vi "Start Module.vi"(8 "error in (no error)":errorcluster, 10 "Config Section":string, 11 "Run as Singleton? (F)":bool) -> (0 "error out":errorcluster, 1 "Wait for Event Sync?":bool, 2 "DB_CONNECTOR Broadcast Events":T1, 3 "Module ID":i32)   [LabVIEW 2014, in "DB_CONNECTOR.lvlib"]
doc: "Launches the Module Main.vi.\n_____\nBased on Delacor QMH Project Template 4.0.0.43."
uses:
  DB_CONNECTOR.lvlib
  Broadcast Events--cluster.ctl
  Did Init Argument--cluster.ctl
  Status Updated Argument--cluster.ctl
  Error Reported Argument--cluster.ctl
  Stop Argument--cluster.ctl
  Get Module Execution Status Argument--cluster.ctl
  Fast Query Reply Argument--cluster.ctl
  Module Running State--enum.ctl
  <vilib>/Delacor/Delacor QMH/Libraries/Cloneable Module Admin_class/Delacor_lib_QMH_Cloneable Module Admin.lvclass
  <vilib>/Delacor/Delacor QMH/Libraries/Cloneable Module Admin_class/Delacor_lib_QMH_Cloneable Module Admin.lvclass/Delacor_lib_QMH_Cloneable Module Admin.ctl
  <vilib>/Delacor/Delacor QMH/Libraries/Module Admin_class/Delacor_lib_QMH_Module Admin.lvclass/Delacor_lib_QMH_Module Admin.ctl
  <vilib>/Delacor/Delacor QMH/Libraries/Cloneable Module Admin_class/Delacor_lib_QMH_Set Module ID.vi
  <vilib>/Delacor/Delacor QMH/Libraries/Module Admin_class/Delacor_lib_QMH_Set External Launch.vi
  <vilib>/Utility/error.llb/Error Cluster From Error Code.vi
  <vilib>/ErrorRing/Error Ring.xnode
  Clone Registration/Clone Registration.lvlib
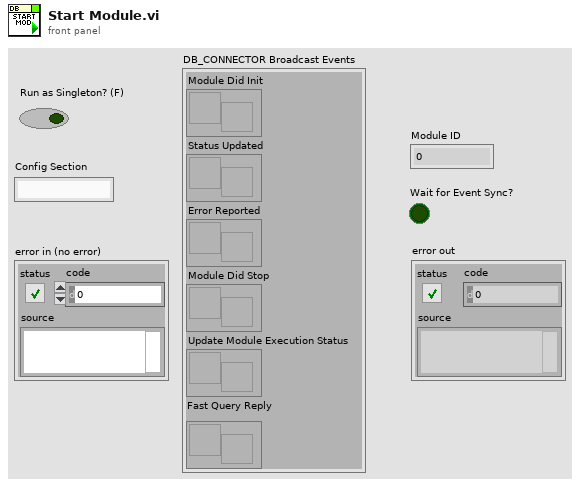
[diagram p1: front panel]
types:
  T1 = typedef "DB_CONNECTOR.lvlib/Broadcast Events--cluster.ctl" = cluster{"Module Did Init":refnum<user-event>, "Status Updated":refnum<user-event>, "Error Reported":refnum<user-event>, "Module Did Stop":refnum<user-event>, "Update Module Execution Status":refnum<user-event>, "Fast Query Reply":refnum<user-event>}
  T2 = typedef "DB_CONNECTOR.lvlib/Module Running State--enum.ctl" = enum16{"Not Running", "Running as Cloneable", "Running as Singleton"}
  T3 = enum32{"Bad", "Idle", "Run top level", "Running"}
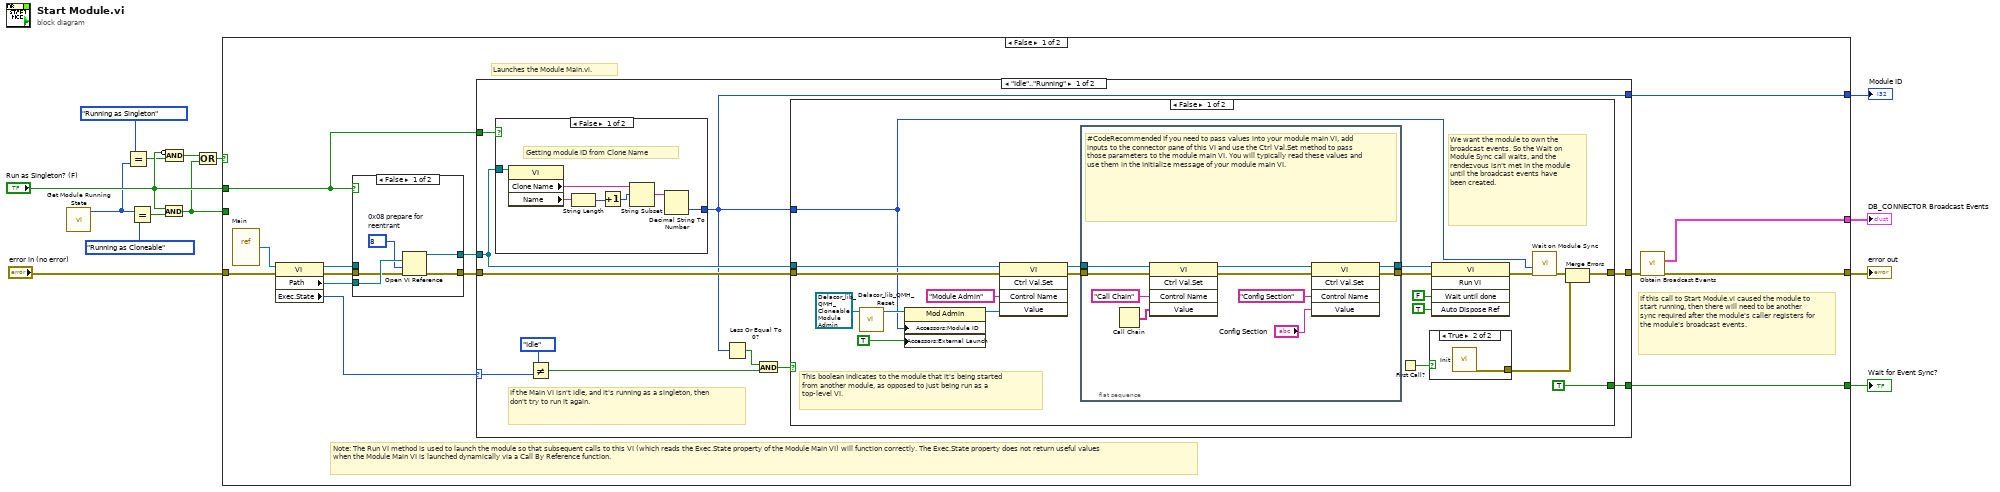
[diagram p0: block diagram]
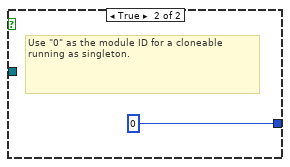
[diagram p3: hidden frame]
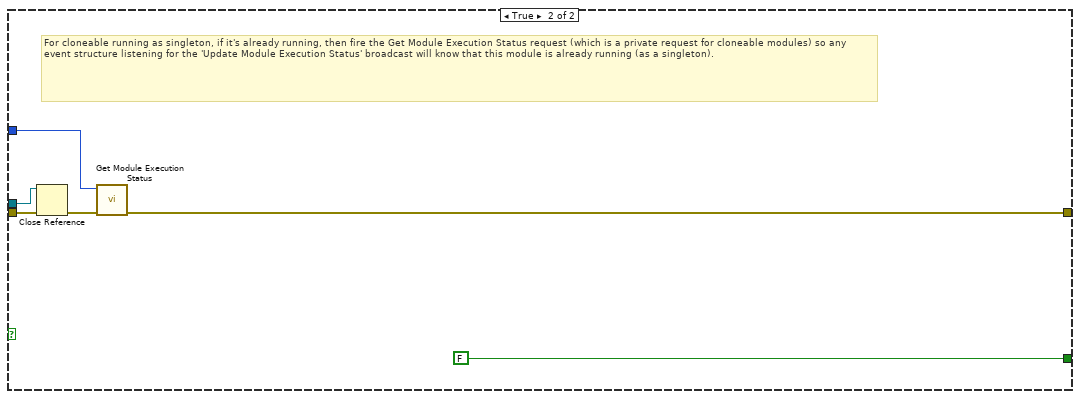
[diagram p5: hidden frame]
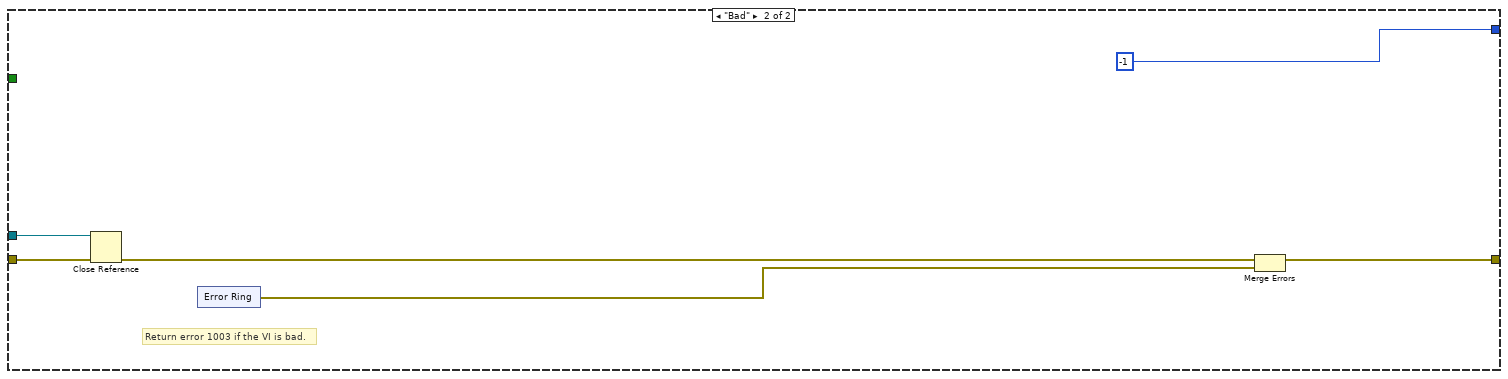
[diagram p6: hidden frame]
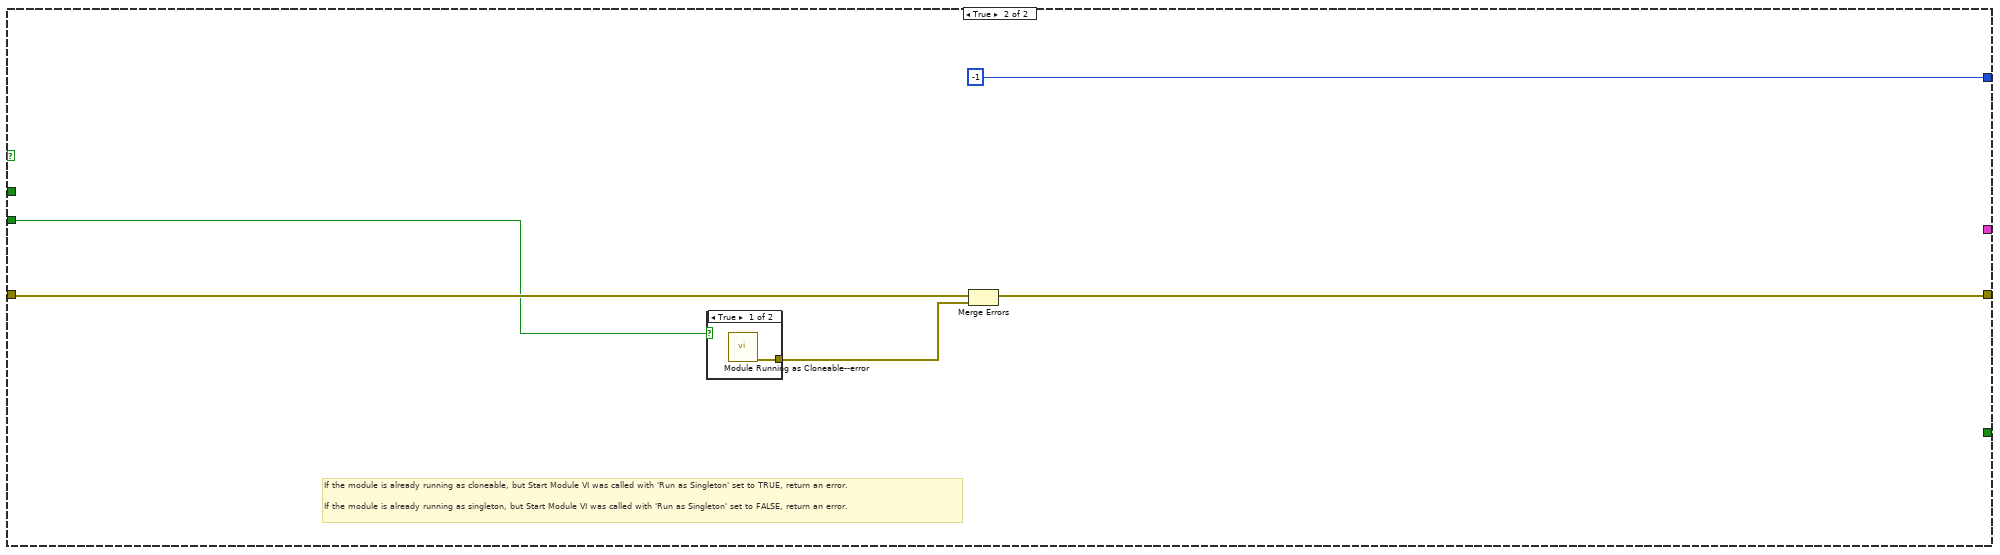
[diagram p7: hidden frame]
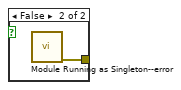
[diagram p8: hidden frame]
diagram:
  n1 = call "Get Module Running State.vi"() -> ("Module Running State"=w3:T2)  [unwired: 11 in]
  n2 = Equal?(x=Module_Running_State--enum."Running as Singleton", y=w3) -> (x = y?=w4:bool)
  n3 = Equal?(x=w3, y=Module_Running_State--enum."Running as Cloneable") -> (x = y?=w8:bool)
  n4 = And(x="Run as Singleton? (F)", y=w8) -> (x .and. y?=w1:bool)
  n5 = Compound Arithmetic op=AND(invert "Run as Singleton? (F)", w4) -> (w6:bool)
  n6 = Or(x=w6, y=w1) -> (x .or. y?=w7:bool)
  n7 = case shown="False" w7 {
    tunnel: "error in (no error)" -> [w28 w106]
    tunnel: [w26 w105] -> w13
    tunnel: [w25 _] -> w12
    tunnel: [w24 _] -> w11
    tunnel: [w20 -1] -> w10
    tunnel: "Run as Singleton? (F)" -> [w16 _]
    tunnel: w1 -> [_ w102]
    frame False {
      # "Note: The Run VI method is used to launch the module so that subsequent calls to this VI (which reads the Exec.State property of the Module Main VI) will function correctly. The Exec.State property does not return useful values when the Module Main VI is launched dynamically via a Call By Reference function."
      # "If this call to Start Module.vi caused the module to start running, then there will need to be another sync required after the module's caller registers for the module's broadcast events."
      # "Launches the Module Main.vi."
      n8 = vi-ref "Main.vi"() -> (w19:refnum<vi>)
      n9 = property class="VI"(reference=w19, error in=w28) -> (reference out=w15:refnum<vi>, error out=w22:errorcluster, "Path"=w23:path, "Exec.State"=w17:T3)
      n10 = case shown="False" w16 {
        tunnel: w23 -> [w33 _]
        tunnel: w22 -> [w32 w35]
        tunnel: [w31 w35] -> w21
        tunnel: [w29 w34] -> w18
        tunnel: w15 -> [_ w34]
        frame False {
          w30 = 8  # 0x08 prepare for reentrant
          n11 = Open VI Reference(vi path=w33, options=w30, error in (no error)=w32) -> (vi reference=w29:refnum<vi>, error out=w31:errorcluster)  [unwired: 3 in]
        }
        frame True {
        }
      }
      n12 = case shown="\"Idle\"..\"Running\"" w17 {
        selector: w17 -> [w42 _]
        tunnel: w21 -> [w46 w97]
        tunnel: w18 -> [w44 w96]
        tunnel: [w43 w94] -> w27
        tunnel: [w45 _] -> w24
        tunnel: [w37 -1] -> w20
        tunnel: w16 -> [w36 _]
        frame "Idle".."Running" {
          # "If the Main VI isn't idle, and it's running as a singleton, then don't try to run it again."
          n13 = case shown="False" w36 {
            tunnel: w44 -> [w53 _]
            tunnel: [w47 0] -> w37
            frame False {
              # "Getting module ID from Clone Name"
              n14 = property class="VI"(reference=w53) -> ("Clone Name"=w50:string, "Name"=w49:string)  [unwired: 1 in, 2 out]
              n15 = String Length(string=w49) -> (length=w51:i32)
              n16 = Increment(x=w51) -> (x+1=w52:i32)
              n17 = String Subset ("Getting module ID from Clone Name")(string=w50, offset (0)=w52) -> (substring=w48:string)  [unwired: 1 in]
              n18 = Decimal String To Number(string=w48) -> (number=w47:i32)  [unwired: 2 in, 1 out]
            }
            frame True {
              # "Use \"0\" as the module ID for a cloneable running as singleton."
            }
          }
          n19 = Not Equal?(x=T3."Idle", y=w42) -> (x != y?=w40:bool)
          n20 = Less Or Equal To 0?(x=w37) -> (x <= 0?=w38:bool)
          n21 = And(x=w38, y=w40) -> (x .and. y?=w39:bool)
          n22 = case shown="False" w39 {
            tunnel: w46 -> [w74 w90]
            tunnel: [TRUE FALSE] -> w45
            tunnel: w44 -> [w67 w87]
            tunnel: [w65 w86] -> w43
            tunnel: w37 -> [w59 w89]
            frame False {
              # "We want the module to own the broadcast events. So the Wait on Module Sync call waits, and the rendezvous isn't met in the module until the broadcast events have been created."
              # "This boolean indicates to the module that it's being started from another module, as opposed to just being run as a top-level VI."
              n23 = call-dynamic "Delacor_lib_QMH_Reset.vi"("Mod Admin in"=refnum<class "Delacor_lib_QMH_Cloneable Module Admin.lvclass"> refnum) -> ("Mod Admin out"=w63:refnum<class "Delacor_lib_QMH_Cloneable Module Admin.lvclass">)  [unwired: 9 in, 1 out]
              n24 = property class="Mod Admin"(reference=w63, "Accessors:Module ID"=w59, "Accessors:External Launch"=TRUE) -> (reference out=w62:refnum<class "Delacor_lib_QMH_Cloneable Module Admin.lvclass">)  [unwired: 1 in, 1 out]
              n25 = invoke class="VI" method="Ctrl Val.Set"(reference=w67, error in=w74, "Control Name"="Module Admin", "Value"=w62) -> (reference out=w58:refnum<vi>, error out=w57:errorcluster)  [unwired: 1 in, 3 out]
              n26 = flat-sequence {
                tunnel: w58 -> [w83]
                tunnel: [w77] -> w56
                tunnel: w57 -> [w82]
                tunnel: [w78] -> w55
                frame #0 {
                  # "#CodeRecommended If you need to pass values into your module main VI, add inputs to the connector pane of this VI and use the Ctrl Val.Set method to pass those parameters to the module main VI. You will typically read these values and use them in the Initialize message of your module main VI."
                  n27 = Call Chain() -> (call chain=w81:string[])
                  n28 = invoke class="VI" method="Ctrl Val.Set"(reference=w83, error in=w82, "Control Name"="Call Chain", "Value"=w81) -> (reference out=w79:refnum<vi>, error out=w80:errorcluster)  [unwired: 1 in, 3 out]
                  n29 = invoke class="VI" method="Ctrl Val.Set"(reference=w79, error in=w80, "Control Name"="Config Section", "Value"="Config Section") -> (reference out=w77:refnum<vi>, error out=w78:errorcluster)  [unwired: 1 in, 3 out]
                }
              }
              n30 = First Call?() -> (First Call?: T/F=w66:bool)
              n31 = case shown="True" w66 {
                tunnel: [_ w85] -> w64
                frame False {
                }
                frame True {
                  n32 = call "Init.vi"() -> ("error out"=w85:errorcluster)  [unwired: 8 in, 3 out]
                }
              }
              n33 = invoke class="VI" method="Run VI"(reference=w56, error in=w55, "Wait until done"=FALSE ("Wait Until Done"), "Auto Dispose Ref"=TRUE ("Auto Dispose Reference")) -> (error out=w71:errorcluster)  [unwired: 1 in, 4 out]
              n34 = call "Wait on Module Sync.vi"("error in (no error)"=w71, "Module ID"=w59) -> ("error out"=w70:errorcluster)  [unwired: 9 in]
              n35 = Merge Errors(w70, w64) -> (w65:errorcluster)
            }
            frame True {
              # "For cloneable running as singleton, if it's already running, then fire the Get Module Execution Status request (which is a private request for cloneable modules) so any event structure listening for the 'Update Module Execution Status' broadcast will know that this module is already running (as a singleton)."
              n36 = Close Reference(reference=w87, error in (no error)=w90) -> (error out=w88:errorcluster)
              n37 = call "Get Module Execution Status.vi"("error in (no error)"=w88, "Module ID"=w89) -> ("error out"=w86:errorcluster)  [unwired: 9 in]
            }
          }
        }
        frame "Bad" {
          # "Return error 1003 if the VI is bad."
          n38 = Close Reference(reference=w96, error in (no error)=w97) -> (error out=w95:errorcluster)
          n39 = xnode "Error Ring"() -> ("error out"=w93:errorcluster)
          n40 = Merge Errors(w95, w93) -> (w94:errorcluster)
        }
      }
      n41 = call "Obtain Broadcast Events.vi"("error in (no error)"=w27) -> ("error out"=w26:errorcluster, "DB_CONNECTOR Broadcast Events"=w25:T1)  [unwired: 9 in]
    }
    frame True {
      # "If the module is already running as cloneable, but Start Module VI was called with 'Run as Singleton' set to TRUE, return an error.\n\nIf the module is already running as singleton, but Start Module VI was called with 'Run as Singleton' set to FALSE, return an error."
      n42 = case shown="True" w102 {
        tunnel: [w107 w108] -> w103
        frame True {
          n43 = call "Module Running as Cloneable--error.vi"() -> ("error out"=w107:errorcluster)  [unwired: 11 in]
        }
        frame False {
          n44 = call "Module Running as Singleton--error.vi"() -> ("error out"=w108:errorcluster)  [unwired: 11 in]
        }
      }
      n45 = Merge Errors(w106, w103) -> (w105:errorcluster)
    }
  }
  "error out" <- w13
  "DB_CONNECTOR Broadcast Events" <- w12
  "Wait for Event Sync?" <- w11
  "Module ID" <- w10
